vi "P31_Count3.vi"() -> ()   [LabVIEW 2022 SP3]
uses:
  <vilib>/MakerHub/LINX/Private/Type Defs/Seven Segment Control.ctl
  <vilib>/MakerHub/LINX/Public/Peripherals/Digital/Digital Read 1 Chan.vi
  <vilib>/MakerHub/LINX/Public/Peripherals/Digital/Digital Read N Chans.vi
  <vilib>/MakerHub/LINX/Private/Local IO/LinxDigitalRead.vi
  <vilib>/MakerHub/LINX/Public/Utilities/Check Channel.vi
  <vilib>/MakerHub/LINX/Public/Utilities/Open Serial.vi
  <vilib>/MakerHub/LINX/Private/Utilties/Generate Error.vi
  <vilib>/MakerHub/LINX/LMH-LINX.lvlib
panel:
  out "Seven Seg Indicator 3":T1
  out "Seven Seg Indicator 2":T1
  out "Seven Seg Indicator":T1
  in  "Serial Port":refnum<visa-resource-name>
  in  "rst":bool
  in  "RESET":bool
  in  "B2":bool
  in  "UP":bool
  in  "stop":bool
  out "Numeric":dbl
  in  "s/s":bool
  in  "START / STOP":bool
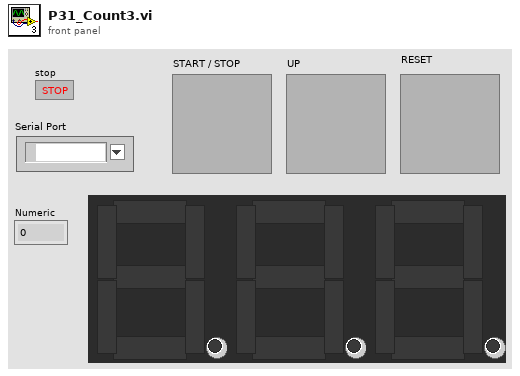
[diagram p1: front panel]
types:
  T1 = typedef "LMH-LINX.lvlib/Seven Segment Control.ctl" = cluster{"Segment 0":bool, "Segment 1":bool, "Segment 2":bool, "Segment 3":bool, "Segment 4":bool, "Segment 5":bool, "Segment 6":bool, "DP":bool}
  T2 = typedef "LMH-LINX.lvlib/LINX Ref.ctl" = cluster{"IO":T3, "Interface":T4, "LINX Device Config":T5}
  T3 = typedef "LMH-LINX.lvlib/Platform.ctl" = enum16{"Remote", "Local"}
  T4 = typedef "LMH-LINX.lvlib/Interface.ctl" = enum16{"Serial", "TCP"}
  T5 = typedef "LMH-LINX.lvlib/Device.lvlib/LINX Device Config.ctl" = cluster{"Interface":T4, "COM Port":refnum<visa-resource-name>, "TCP Configuration":T6, "Device Family":u8, "Device ID":u8, "Device Name":string, "TCP Ref":refnum<k5>, "Channels":T7}
  T6 = typedef "LMH-LINX.lvlib/Device.lvlib/TCP Config.ctl" = cluster{"IP Address":string, "Port":u16}
  T7 = typedef "LMH-LINX.lvlib/Channels.ctl" = cluster{"DI":u8[], "DO":u8[], "AI":u8[], "AO":u8[], "PWM":u8[], "QE":u8[], "UART":u8[], "I2C 2":u8[], "SPI":u8[], "CAN":u8[], "Servo":u8[], "AI Ref (V)":dbl, "AI Resolution (Bits)":u8, "AO Ref (V)":dbl, "AO Resolution (Bits)":u8}
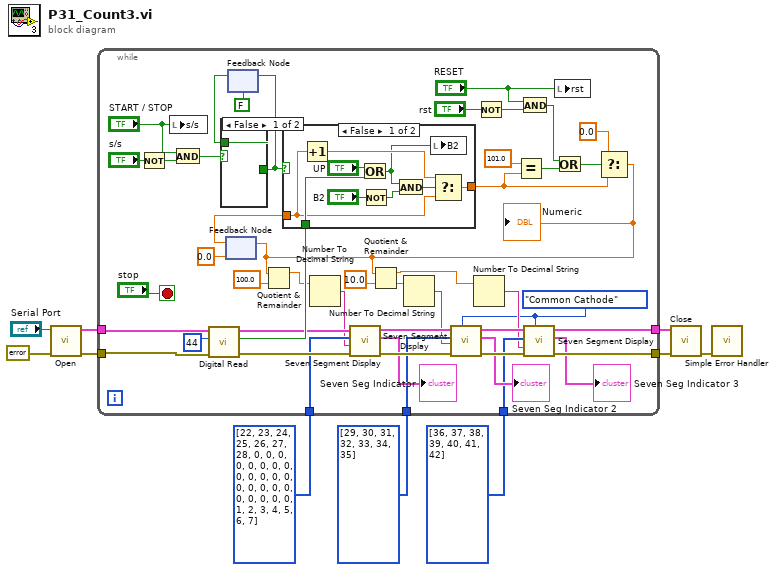
[diagram p0: block diagram]
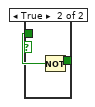
[diagram p2: hidden frame]
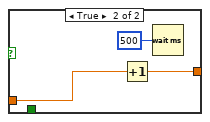
[diagram p3: hidden frame]
diagram:
  n1 = call-poly <vilib>:"Open.vi"("Error In"=errorcluster {"status"=FALSE, "code"=0, "source"=""}, "Serial Port"="Serial Port") -> ("Error Out"=w4:errorcluster, "LINX Resource"=w8:T2)  [unwired: 7 in, 1 out]
  n2 = while {
    tunnel: w8 -> [w42]
    tunnel: w4 -> [w41]
    tunnel: [w32] -> w6
    tunnel: [w31] -> w5
    tunnel: u8[] [22, 23, 24, 25, 26, 27, 28, 0, 0, 0, 0, 0, 0, 0, 0, 0, 0, 0, 0, 0, 0, 0, 0, 0, 0, 0, 0, 0, 0, 0, 1, 2, 3, 4, 5, 6, 7] ("Channels") -> [w27]
    tunnel: u8[] [29, 30, 31, 32, 33, 34, 35] ("Channels") -> [w26]
    tunnel: u8[] [36, 37, 38, 39, 40, 41, 42] ("Channels") -> [w25]
    stop <- "stop" stop-if-true
    w18 = enum16{"Common Anode", "Common Cathode"}."Common Cathode" ("Seven Seg Type (Common Anode)")
    n3 = Not(x="s/s") -> (.not. x?=w57:bool)
    n4 = local write "s/s"("START / STOP") -> ()
    n5 = And(x="START / STOP", y=w57) -> (x .and. y?=w52:bool)
    n6 = call-poly <vilib>:"Digital Read.vi"("Error In"=w41, "DI Channel"=u8 44, "LINX Resource"=w42) -> ("Error Out"=w37:errorcluster, "DI Value"=w39:bool, "LINX Resource"=w38:T2)  [unwired: 6 in]
    n7 = feedback #1(0.0) -> (w55:dbl)
    n8 = feedback #2(FALSE) -> (w51:bool)
    n9 = case shown="False" w52 {
      tunnel: [w58 w60] -> w50
      tunnel: w51 -> [w58 w59]
      frame False {
      }
      frame True {
        n10 = Not(x=w59) -> (.not. x?=w60:bool)
      }
    }
    n11 = feedback-in #2(w50) -> ()
    n12 = case shown="False" w50 {
      tunnel: [w68 w70] -> w11
      tunnel: w55 -> [w61 w71]
      tunnel: w39 -> [w62 _]
      frame False {
        n13 = Increment(x=w61) -> (x+1=w69:dbl)
        n14 = Or(x="UP", y=w62) -> (x .or. y?=w63:bool)
        n15 = Not(x="B2") -> (.not. x?=w66:bool)
        n16 = And(x=w63, y=w66) -> (x .and. y?=w65:bool)
        n17 = local write "B2"(w63) -> ()
        n18 = Select(t=w69, s=w65, f=w61) -> (s? t:f=w68:dbl)
      }
      frame True {
        n19 = Increment(x=w71) -> (x+1=w70:dbl)
        n20 = Wait (ms)(milliseconds to wait=u32 500) -> ()  [unwired: 1 out]
      }
    }
    n21 = Not(x="rst") -> (.not. x?=w44:bool)
    n22 = Equal?(x=101.0, y=w11) -> (x = y?=w47:bool)
    n23 = And(x="RESET", y=w44) -> (x .and. y?=w43:bool)
    n24 = local write "rst"("RESET") -> ()
    n25 = Or(x=w43, y=w47) -> (x .or. y?=w46:bool)
    n26 = Select(t=0.0, s=w46, f=w11) -> (s? t:f=w20:dbl)
    "Numeric" <- w20
    n27 = feedback-in #1(w20) -> ()
    n28 = Quotient & Remainder(x=w20, y=100.0) -> (x-y*floor(x/y)=w16:dbl)  [unwired: 1 out]
    n29 = Number To Decimal String(number=w16) -> (decimal integer string=w24:string)  [unwired: 1 in]
    n30 = call <vilib>:"Seven Segment Display.vi"("Error In"=w37, "Character"=w24, "Channels"=w27, "LINX Resource"=w38) -> ("Error Out"=w34:errorcluster, "Seven Seg Indicator"=→"Seven Seg Indicator":T1, "LINX Resource"=w36:T2)  [unwired: 5 in]
    n31 = Quotient & Remainder(x=w20, y=10.0) -> (x-y*floor(x/y)=w15:dbl, floor(x/y)=w17:dbl)
    n32 = Number To Decimal String(number=w17) -> (decimal integer string=w19:string)  [unwired: 1 in]
    n33 = call <vilib>:"Seven Segment Display.vi"("Seven Seg Type (Common Anode)"=w18, "Error In"=w34, "Character"=w19, "Channels"=w26, "LINX Resource"=w36) -> ("Error Out"=w33:errorcluster, "Seven Seg Indicator"=→"Seven Seg Indicator 2":T1, "LINX Resource"=w35:T2)  [unwired: 4 in]
    n34 = Number To Decimal String(number=w15) -> (decimal integer string=w22:string)  [unwired: 1 in]
    n35 = call <vilib>:"Seven Segment Display.vi"("Seven Seg Type (Common Anode)"=w18, "Error In"=w33, "Character"=w22, "Channels"=w25, "LINX Resource"=w35) -> ("Error Out"=w32:errorcluster, "Seven Seg Indicator"=→"Seven Seg Indicator 3":T1, "LINX Resource"=w31:T2)  [unwired: 4 in]
  }
  n36 = call <vilib>:"Close.vi"("Error In"=w6, "LINX Resource"=w5) -> ("Error Out"=w7:errorcluster)  [unwired: 9 in]
  n37 = call <vilib>:"Simple Error Handler.vi"("error in (no error)"=w7) -> ()  [unwired: 4 in, 5 out]
